vi "LogTX.vi"(8 "error in (no error)":errorcluster, 11 "Server in":refnum<class "Server.lvclass">) -> (0 "error out":errorcluster, 3 "Server out":refnum<class "Server.lvclass">)   [LabVIEW 2018]
uses:
  Server.lvclass
  Comm/Comm.lvclass
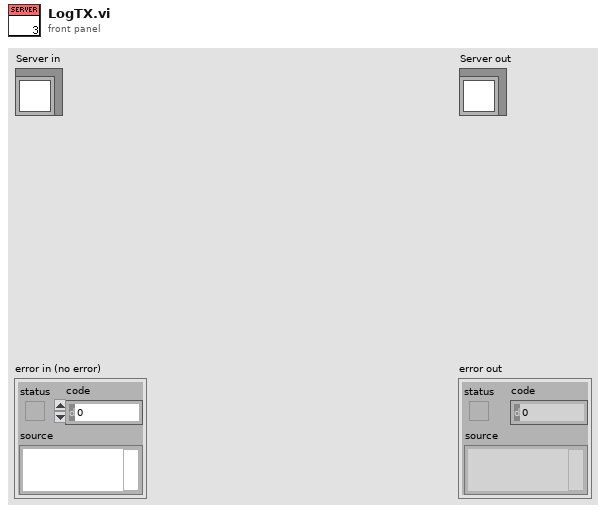
[diagram p1: front panel]
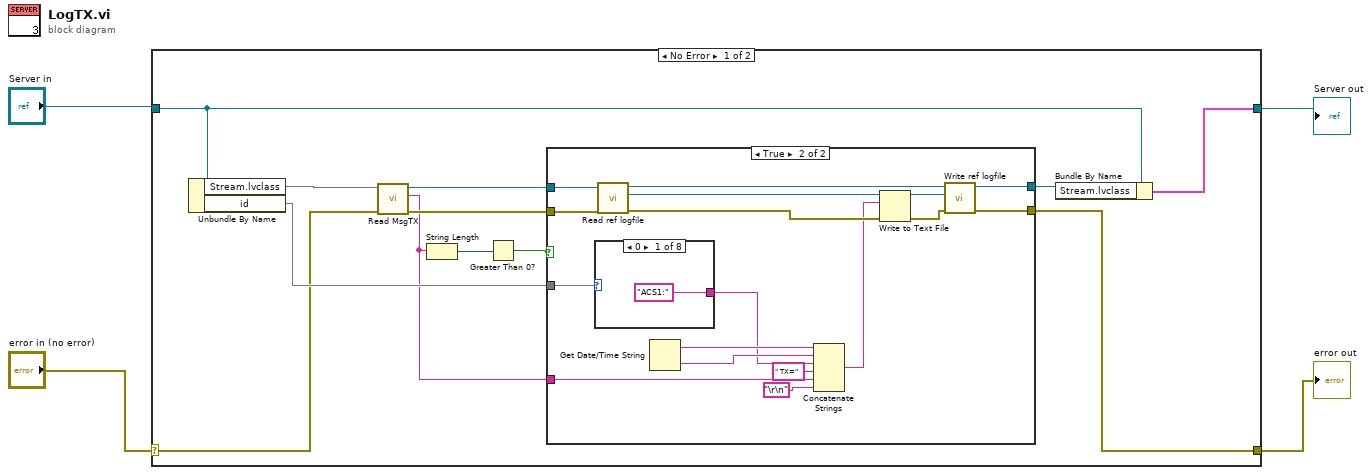
[diagram p0: block diagram]
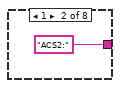
[diagram p3: hidden frame]
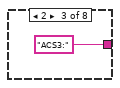
[diagram p4: hidden frame]
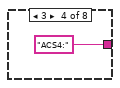
[diagram p5: hidden frame]
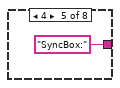
[diagram p6: hidden frame]
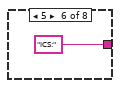
[diagram p7: hidden frame]
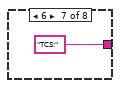
[diagram p8: hidden frame]
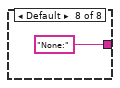
[diagram p9: hidden frame]
diagram:
  n1 = case shown="No Error" "error in (no error)" {
    selector: "error in (no error)" -> [w7 w45]
    tunnel: [w8 w45] -> w1
    tunnel: [w9 w44] -> w2
    tunnel: "Server in" -> [w11 w44]
    frame No Error {
      n2 = Unbundle By Name(w11) -> ("Stream.lvclass"=w6, "id"=w16)
      n3 = call-dynamic "Read MsgTX.vi"("error in (no error)"=w7, "Comm in"=w6) -> ("error out"=w13:errorcluster, "MsgTX"=w12:string, "Comm out"=w15:refnum<class "Comm.lvclass">)  [unwired: 7 in]
      n4 = String Length(string=w12) -> (length=w5:i32)
      n5 = Greater Than 0?(x=w5) -> (x > 0?=w14:bool)
      n6 = case shown="True" w14 {
        tunnel: w16 -> [_ w34]
        tunnel: w15 -> [w18 w30]
        tunnel: w13 -> [w17 w29]
        tunnel: w12 -> [_ w26]
        tunnel: [w17 w20] -> w8
        tunnel: [w18 w19] -> w10
        frame False {
        }
        frame True {
          n7 = case shown="0" w34 {
            tunnel: ["ACS1:" "ACS2:" "ACS3:" "ACS4:" "SyncBox:" "ICS:" "TCS:" "None:"] -> w31
            frame 0 {
            }
            frame 1 {
            }
            frame 2 {
            }
            frame 3 {
            }
            frame 4 {
            }
            frame 5 {
            }
            frame 6 {
            }
            frame Default {
            }
          }
          n8 = call-dynamic "Read ref logfile.vi"("error in (no error)"=w29, "Comm in"=w30) -> ("error out"=w28:errorcluster, "ref logfile"=w35:refnum<file>, "Comm out"=w22:refnum<class "Comm.lvclass">)  [unwired: 7 in]
          n9 = Get Date/Time String() -> (date string=w33:string, time string=w32:string)  [unwired: 3 in]
          n10 = Concatenate Strings(w33, w32, w31, " TX=" ("string"), w26, "\r\n" ("string")) -> (w24:string)
          n11 = Write to Text File(file (use dialog)=w35, text=w24, error in=w28) -> (refnum out=w23:refnum<file>, error out=w21:errorcluster)  [unwired: 1 in, 1 out]
          n12 = call-dynamic "Write ref logfile.vi"("error in (no error)"=w21, "ref logfile"=w23, "Comm in"=w22) -> ("error out"=w20:errorcluster, "Comm out"=w19:refnum<class "Comm.lvclass">)  [unwired: 7 in]
        }
      }
      n13 = Bundle By Name(cluster=w11, "Stream.lvclass"=w10) -> (w9:cluster{})
    }
    frame Error {
    }
  }
  "error out" <- w1
  "Server out" <- w2
